vi "Thermocouple - Thermal Camera Validation.vi"() -> ()   [LabVIEW 2024]
doc: "This example demonstrates how to continuously acquire thermocouple measurements using a DAQmx device.\n\nFor instructions on how to connect your signals to the DAQ device, refer to your device documentation."
uses:
  <vilib>/Utility/error.llb/DialogType.ctl
  <vilib>/DAQmx/read.llb/DAQmx Read (Analog 1D Wfm NChan 1Samp).vi
  <vilib>/DAQmx/create/channels.llb/DAQmx Create Channel (AI-Temperature-Thermocouple).vi
  <vilib>/DAQmx/miscellaneous.llb/DAQmx Fill In Error Info.vi
  <resource>/objmgr/daqmx.rc
panel:
  in  "Log File":path
  out "resulting string":string
  out "Y":dbl[](array[numeric])
  in  "Auto Zero Mode":i32(ring)=10230 items=["None"=10230, "Once"=10244, "Every Sample"=10164]
  in  "CJC Channel":refnum<k21>
  in  "CJC Value":dbl=25.0 format="%0.2f"
  in  "CJC Source":i32(ring)=10116 items=["Built-In"=10200, "Constant Value"=10116, "Channel"=10113]
  in  "Thermocouple Type":i32(ring)=10072 items=["J"=10072, "K"=10073, "N"=10077, "R"=10082, "S"=10085, "T"=10086, "B"=10047, "E"=10055, "A"=16208, "C"=16209]
  in  "Units":i32(ring)=10143 items=["Deg C"=10143, "Deg F"=10144, "Kelvins"=10325, "Deg R"=10145, "From Custom Scale"=10065]
  in  "Loop Time (ms)":u32=100
  in  "Stop":bool
  in  "Max Temperature":dbl=100.0
  in  "Min Temperature":dbl
  in  "Physical Channel":tag="Dev1/ai0"
  out "Waveform Chart":waveform(dbl)[](graph)
  # "Acquired Data"
  # "Channel Settings"
  # "Timing Settings"
  # "Auto Zero Settings"
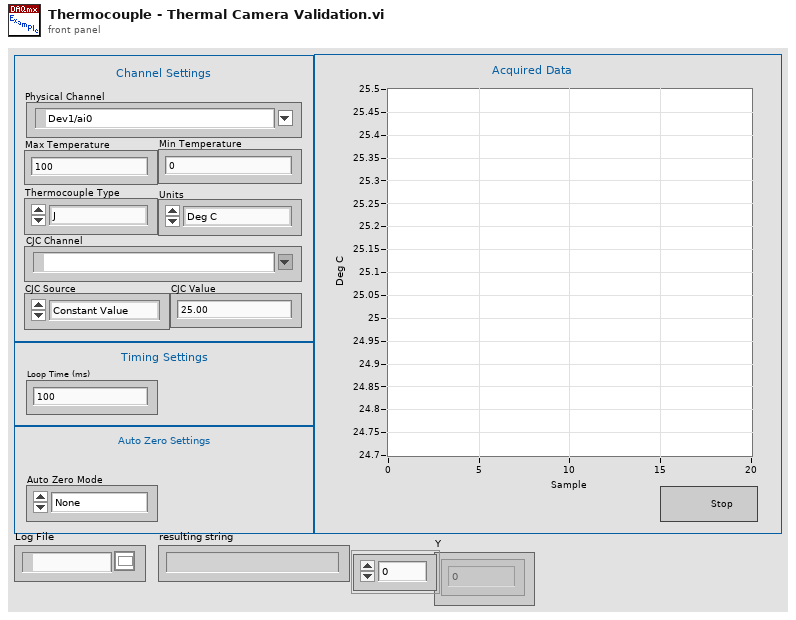
[diagram p1: front panel]
types:
  T1 = enum16{"open", "replace", "create", "open or create", "replace or create", "replace or create with confirmation"}
  T2 = typedef "DialogType.ctl" = u16
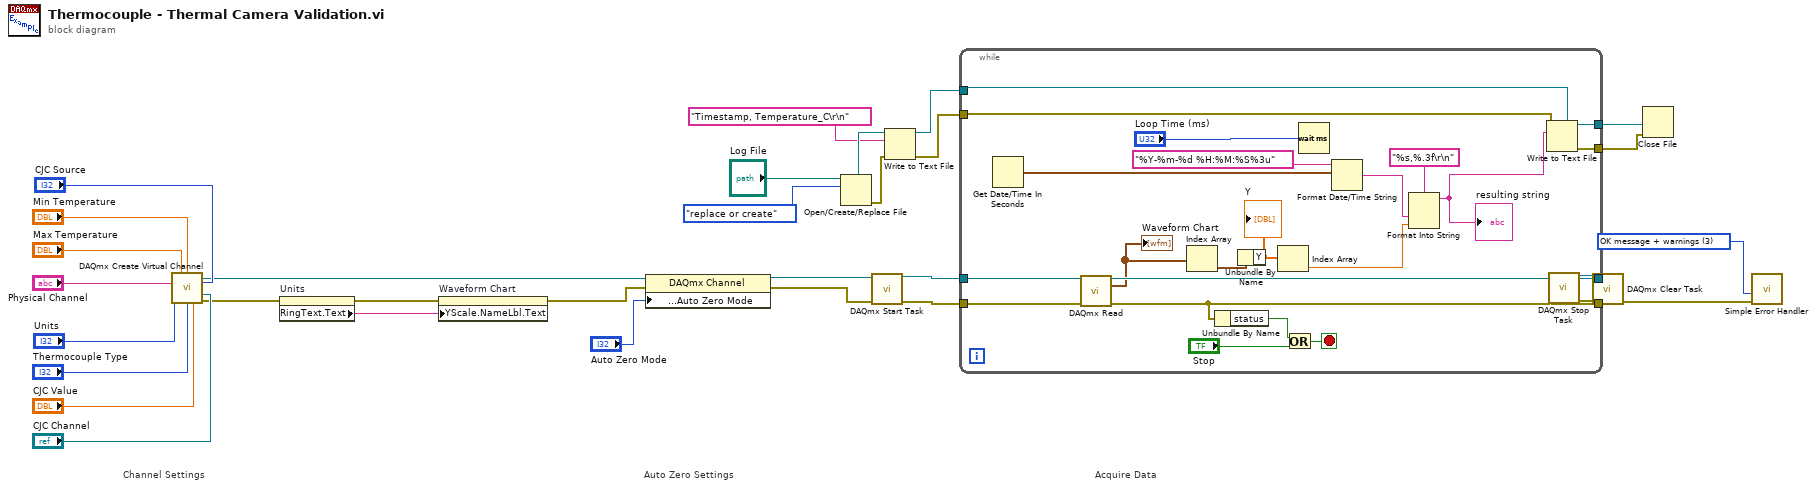
[diagram p0: block diagram]
diagram:
  w10 = T2 3 items=["no dialog", "OK message", "continue or stop message", "OK message + warnings", "continue/stop + warnings"] ("type of dialog (OK msg:1)")
  # "Auto Zero Settings"
  # "Acquire Data"
  # "Channel Settings"
  n1 = call-poly <vilib>:"DAQmx Create Virtual Channel.vi"("maximum value"="Max Temperature", "minimum value"="Min Temperature", "physical channels"="Physical Channel", "cjc source"="CJC Source", "units"="Units", "cjc channel"="CJC Channel", "thermocouple type"="Thermocouple Type", "cjc value"="CJC Value") -> ("task out"=w20:refnum<k21>, "error out"=w22:errorcluster)  [unwired: 6 in]
  n2 = property on="Units" class="Ring (strict)"(error in=w22) -> (error out=w16:errorcluster, "RingText.Text"=w17:string)  [unwired: 1 in, 1 out]
  n3 = property on="Waveform Chart" class="WFChart (strict)"(error in=w16, "YScale.NameLbl.Text"=w17) -> (error out=w15:errorcluster)  [unwired: 1 in, 1 out]
  n4 = property class="DAQmx Channel"(reference=w20, error in=w15, "Analog Input:General Properties:Advanced:High Accuracy Settings:Auto Zero Mode"="Auto Zero Mode") -> (reference out=w19:refnum<k21>, error out=w18:errorcluster)
  n5 = Open/Create/Replace File(file path (use dialog)="Log File", operation (0:open)=T1."replace or create") -> (refnum out=w7:refnum<file>, error out=w2:errorcluster)  [unwired: 4 in, 1 out]
  n6 = call <vilib>:"DAQmx Start Task.vi"("task/channels in"=w19, "error in"=w18) -> ("task out"=w33:refnum<k21>, "error out"=w32:errorcluster)  [unwired: 12 in]
  n7 = Write to Text File(file (use dialog)=w7, text="Timestamp, Temperature_C\r\n", error in=w2) -> (refnum out=w5:refnum<file>, error out=w3:errorcluster)  [unwired: 1 in, 1 out]
  n8 = while {
    tunnel: w33 -> [w54]
    tunnel: w32 -> [w53]
    tunnel: [w50] -> w11
    tunnel: [w51] -> w12
    tunnel: w5 -> [w40]
    tunnel: [w38] -> w4
    tunnel: w3 -> [w37]
    tunnel: [w36] -> w1
    stop <- w52 stop-if-true
    n9 = Get Date/Time In Seconds() -> (seconds since 1Jan1904=w35:timestamp)
    n10 = call-poly <vilib>:"DAQmx Read.vi"("task/channels in"=w54, "error in"=w53) -> ("task out"=w51:refnum<k21>, "data"=w46:waveform(dbl)[], "error out"=w50:errorcluster)  [unwired: 11 in]
    "Waveform Chart" <- w46
    n11 = Index Array(array=w46) -> (element=w45:waveform(dbl))  [unwired: 1 in]
    n12 = Unbundle By Name(w50) -> ("status"=w49:bool)
    n13 = Unbundle By Name(w45) -> ("Y"=w44:dbl[])
    "Y" <- w44
    n14 = Index Array(array=w44) -> (element=w42:dbl)  [unwired: 1 in]
    n15 = Or(x=w49, y="Stop") -> (x .or. y?=w52:bool)
    n16 = Wait (ms)(milliseconds to wait="Loop Time (ms)") -> ()  [unwired: 1 out]
    n17 = Format Date/Time String(time format string (%c)="%Y-%m-%d %H:%M:%S%3u", seconds (now)=w35) -> (date/time string=w41:string)  [unwired: 1 in]
    n18 = Format Into String(format string="%s,%.3f\r\n", w41, w42) -> (resulting string=w39:string)  [unwired: 2 in, 1 out]
    "resulting string" <- w39
    n19 = Write to Text File(file (use dialog)=w40, text=w39, error in=w37) -> (refnum out=w38:refnum<file>, error out=w36:errorcluster)  [unwired: 1 in, 1 out]
  }
  n20 = call <vilib>:"DAQmx Stop Task.vi"("task/channels in"=w12, "error in"=w11) -> ("task out"=w14:refnum<k21>, "error out"=w13:errorcluster)  [unwired: 12 in]
  n21 = call <vilib>:"DAQmx Clear Task.vi"("task in"=w14, "error in"=w13) -> ("error out"=w31:errorcluster)  [unwired: 13 in]
  n22 = Close File(refnum=w4, error in=w1) -> ()  [unwired: 2 out]
  n23 = call <vilib>:"Simple Error Handler.vi"("type of dialog (OK msg:1)"=w10, "error in (no error)"=w31) -> ()  [unwired: 3 in, 5 out]
